vi "Matches.vi"(8 "error in (no error)":errorcluster, 10 "Actual":variant, 11 "IsType in":refnum<class "IsType.lvclass">) -> (0 "error out":errorcluster, 2 "Result":bool, 3 "IsType out":refnum<class "IsType.lvclass">)   [LabVIEW 2017, in "Transparent Assertions.lvlib" / "IsType.lvclass"]
doc: "Evaluates the constraint for <B>Actual</B>. Returns true if the constraint is met."
uses:
  IsType.lvclass
  IsType.lvclass/IsType.ctl
  <vilib>/Utility/Data Type/NI_Data Type.lvlib
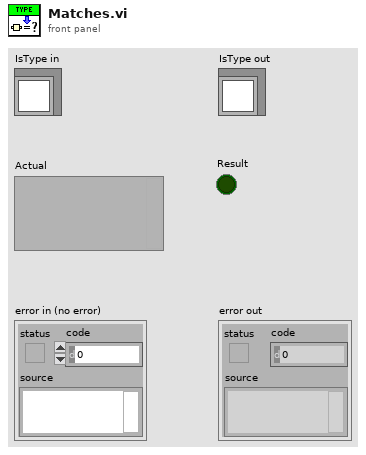
[diagram p1: front panel]
types:
  T1 = typedef "NI_Data Type.lvlib/Data Type.ctl" = enum8{"Invalid Type", "Void", "I8", "I16", "I32", "I64", "U8", "U16", "U32", "U64", "Single Float", "Double Float", "Extended Float", "Single Complex", "Double Complex", "Extended Complex", "Enum U8", "Enum U16", "Enum U32", "Enum U64", "Single Float With Unit", "Double Float With Unit", "Extended Float With Unit", "Single Complex with Unit", "Double Complex with Unit", "Extended Complex with Unit", "Boolean", "String", "Path", "Picture", "Tag", "Array", "Cluster", "Variant", "LV Variant", "Waveform", "Timestamp", "Digital Waveform", "Digital Data", "ExpressData", "Refnum", "External Data", "VI", "Poly VI", "LabVIEW Class Instance", "Fixed Point"}
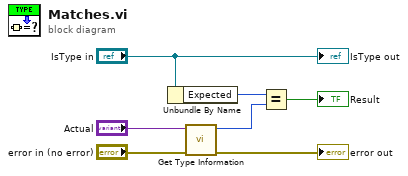
[diagram p0: block diagram]
diagram:
  n1 = Unbundle By Name("IsType in") -> ("Expected"=w3:T1)
  n2 = call <vilib>:"Get Type Information.vi"("error in (no error)"="error in (no error)", "Variant"="Actual") -> ("error out"=→"error out":errorcluster, "Type"=w2:T1)  [unwired: 5 in, 3 out]
  n3 = Equal?(x=w3, y=w2) -> (x = y?=→"Result":bool)
  "IsType out" <- "IsType in"
